vi "Agilent Clean Gain Values.vi"(8 "Error In":errorcluster, 11 "Analog Channels-List":string) -> (0 "Error Out":errorcluster, 3 "String":string)   [LabVIEW 2019]
uses:
  Agilent 34970.lvlib
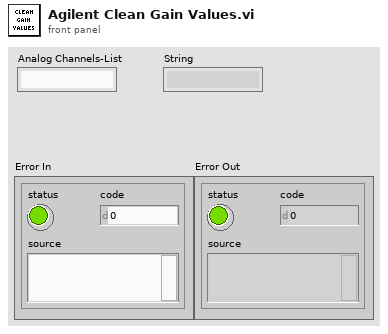
[diagram p1: front panel]
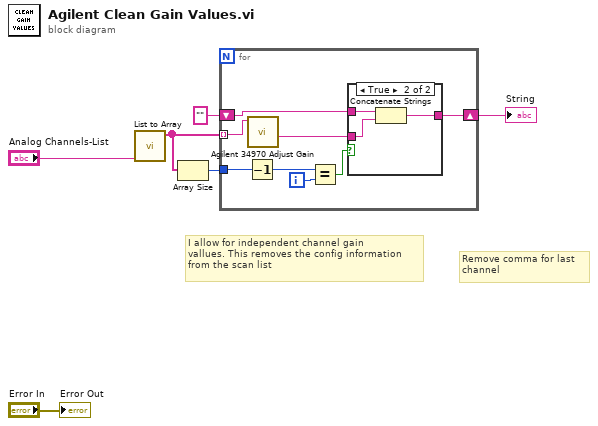
[diagram p0: block diagram]
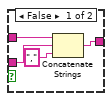
[diagram p2: hidden frame]
diagram:
  # "I allow for independent channel gain\nvallues. This removes the config information\nfrom the scan list"
  # "Remove comma for last\nchannel"
  n1 = call "List to Array.vi"("List (empty)"="Analog Channels-List") -> ("Output String Array"=w4:string[])  [unwired: 9 in, 1 out]
  n2 = Array Size(array=w4) -> (size(s)=w3:i32)
  n3 = for {
    tunnel: w4 -> [w14] mode=indexing
    shift-right: [w12] -> w2
    shift-left: "" -> [w13]
    tunnel: w3 -> [w11]
    i -> [w9]
    n4 = Decrement(x=w11) -> (x-1=w10:i32)
    n5 = call "Agilent 34970 Adjust Gain.vi"("Input Channel"=w14) -> ("Output Channel"=w7:string)  [unwired: 6 in, 4 out]
    n6 = Equal?(x=w10, y=w9) -> (x = y?=w8:bool)
    n7 = case shown="True" w8 {
      tunnel: w13 -> [w18 w21]
      tunnel: w7 -> [w17 w20]
      tunnel: [w15 w19] -> w12
      frame False {
        n8 = Concatenate Strings(w18, w17, "," ("string")) -> (w15:string)
      }
      frame True {
        n9 = Concatenate Strings(w21, w20) -> (w19:string)
      }
    }
  }
  "String" <- w2
  "Error Out" <- "Error In"
